vi "Latch.vi"(7 "Reset":bool, 11 "Input":bool) -> (3 "Output":bool)   [LabVIEW 2012]
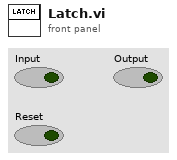
[diagram p1: front panel]
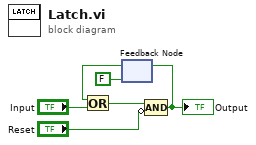
[diagram p0: block diagram]
diagram:
  n1 = feedback #1(FALSE) -> (w3:bool)
  n2 = Or(x=w3, y="Input") -> (x .or. y?=w1:bool)
  n3 = Compound Arithmetic op=AND(w1, invert "Reset") -> (w4:bool)
  "Output" <- w4
  n4 = feedback-in #1(w4) -> ()
